vi "ControlMotorFindZeroEdge.vi"(2 "错误输入":errorcluster, 3 "控制电机":T1) -> (0 "错误输出":errorcluster)   [LabVIEW 2018]
panel:
  out "function return":i32
  out "搜零参数.搜零低速度":dbl
  out "搜零参数.搜零高速度":dbl
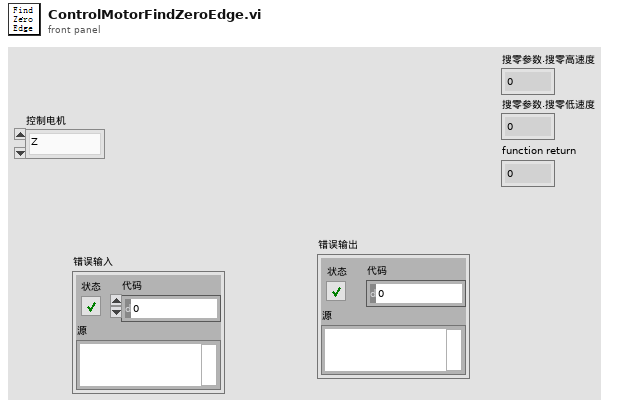
[diagram p1: front panel]
types:
  T1 = typedef "控制电机枚举器.ctl" = enum16{"Z", "Y", "X", "发散角", "俯仰", "旋转"}
  T2 = cluster{"是否停止":enum16{"解除停止", "停止"}, "发生错误停止运行":enum16{"不停止", "停止"}, "发生错误退出运行":enum16{"不退出", "退出"}, "有效电平":cluster{"脉冲信号有效电平":enum16{"低电平有效", "高电平有效"}, "方向信号有效电平 ":enum16{"低电平有效", "高电平有效"}}, "运行脉宽":i32, "加速度和速度边界":cluster{"加速度最大":i32, "速度最大":i32}, "硬件限位设置":cluster{"正限位使能":enum16{"不使能", "使能"}, "正限位极性":enum16{"低电平有效", "高电平有效"}, "负限位使能 ":enum16{"不使能", "使能"}, "负限位极性 ":enum16{"低电平有效", "高电平有效"}}, "伺服报警":cluster{"伺服报警使能":enum16{"不使能", "使能"}, "伺服报警极性":enum16{"低电平有效", "高电平有效"}}, "电机使能":enum16{"不使能", "使能"}, "输出极性":cluster{"寄存器":u32, " fifo":u32, "Bit":u32, "输出极性控制":enum16{"脉冲+方向", "正负脉冲"}}, "运动模式":enum16{"普通模式", "跟踪模式"}, "加速度 puls/s2":i32, "运动速度":cluster{"峰值速度 puls/s":i32, "起始速度puls/s":i32}, "电机速度归一化常量":dbl, "编码器":cluster{"编码器计数模式":enum16{"正交模式", "脉冲+方向模式"}, "编码器计数方向":enum16{"B相超前A相", "A相超前B相"}, "编码器使能":enum16{"不使能", "使能"}, "寄存器位置":i32, "fifo":i32, "data":i32}, "搜零参数":cluster{"orgSW零点开关":enum16{"0开关作为0点", "正限位作为0点", "负限位作为0点"}, "搜零方向":enum16{"正方向", "负方向"}, "零点停止方式":enum16{"立即停止", "减速停止"}, "原点信号边沿":enum16{"下降沿", "上升沿"}, "判断原点位置方向":enum16{"正方向移动", "负方向移动"}, " reducer搜零方式":enum16{"没有减速装置", "原点边缘作为减速", "探针开关作为减速"}, "零点位置":dbl, "搜零高速度":dbl, "搜零低速度":dbl, " 是否等待结束":enum16{"不等待", "等待"}, "编码器索引信号极性":enum16{"下降沿有效", "上升沿有效"}}}
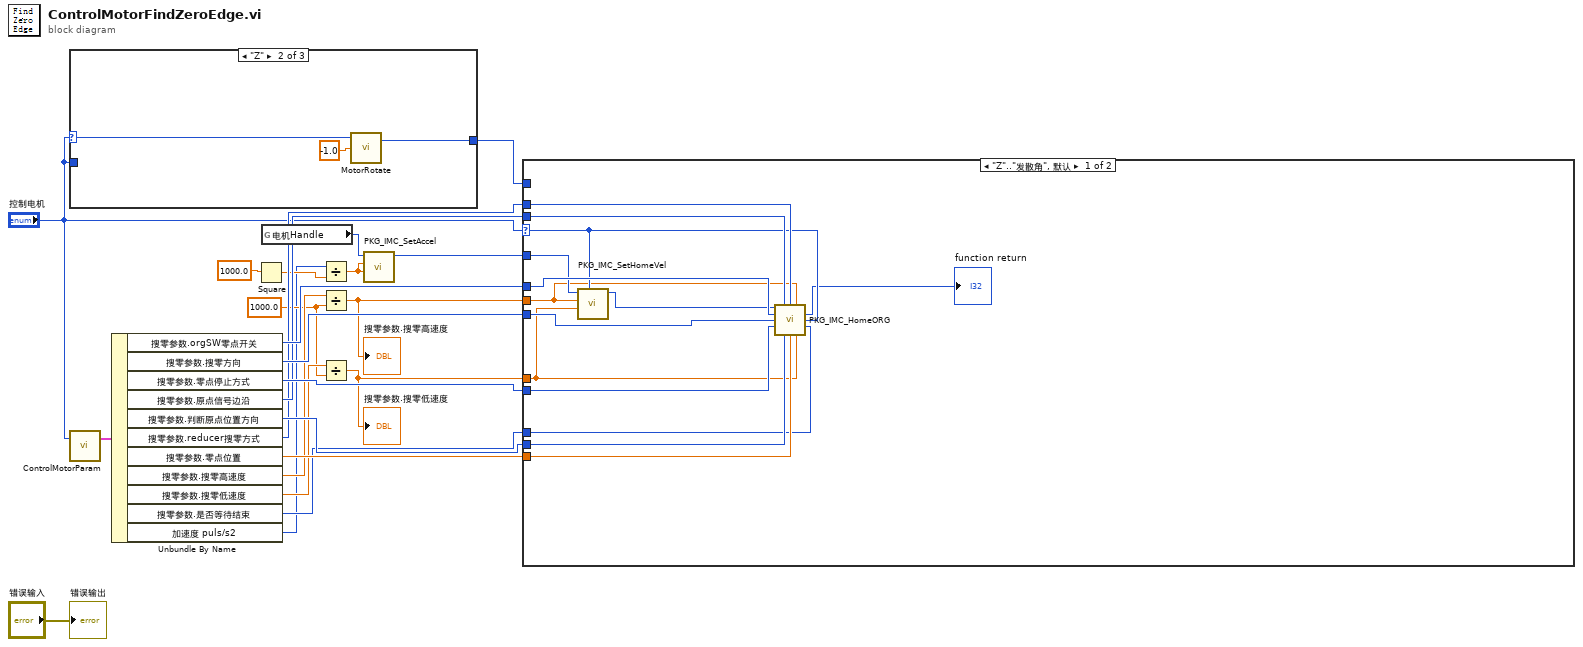
[diagram p0: block diagram]
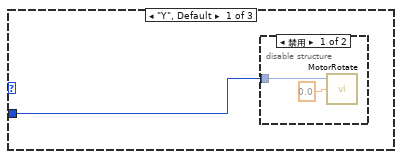
[diagram p2: hidden frame]
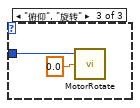
[diagram p4: hidden frame]
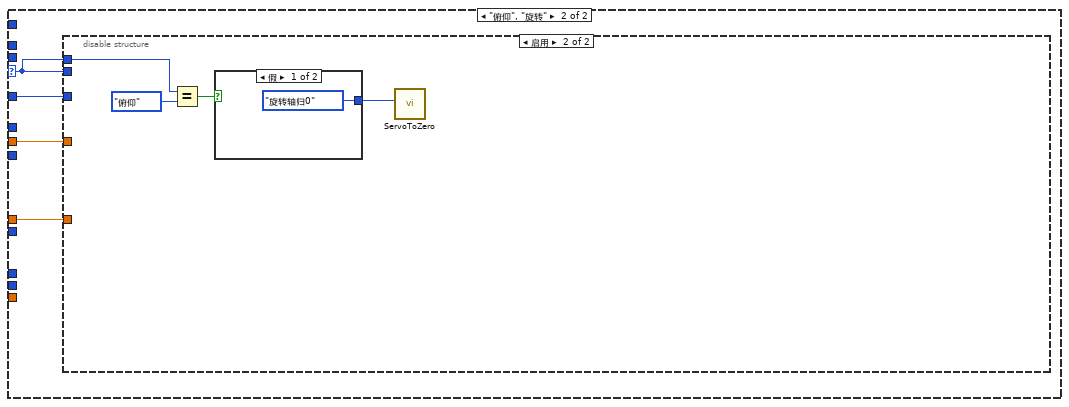
[diagram p5: hidden frame]
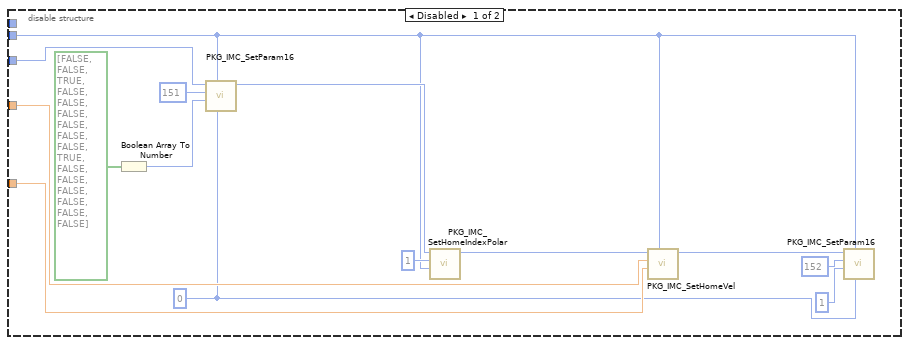
[diagram p6: hidden frame]
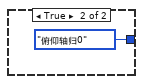
[diagram p7: hidden frame]
diagram:
  w8 = 1000.0 ("y")
  n1 = case shown="\"Z\"" "控制电机" {
    selector: "控制电机" -> [_ w29 _]
    tunnel: "控制电机" -> [w24 _ w30]
    tunnel: [_ w27 _] -> w7
    frame "Y", Default {
      n2 = disable-structure shown="禁用" {
        disable-tunnel: w24 -> [w25 _]
        frame Disabled {
          n3 = call "MotorRotate.vi"("位置"=0.0, "控制电机"=w25) -> ()  [unwired: 2 in, 1 out]
        }
        frame Enabled {
        }
      }
    }
    frame "Z" {
      n4 = call "MotorRotate.vi"("位置"=-1.0, "控制电机"=w29) -> ("返回"=w27:i32)  [unwired: 2 in]
    }
    frame "俯仰", "旋转" {
      n5 = call "MotorRotate.vi"("位置"=0.0, "控制电机"=w30) -> ()  [unwired: 2 in, 1 out]
    }
  }
  n6 = call "ControlMotorParam.vi"("控制电机"="控制电机") -> ("轴参数"=w11:T2)  [unwired: 2 in]
  n7 = Unbundle By Name(w11) -> ("搜零参数.orgSW零点开关"=w23:enum16{"0开关作为0点", "正限位作为0点", "负限位作为0点"}, "搜零参数.搜零方向"=w22:enum16{"正方向", "负方向"}, "搜零参数.零点停止方式"=w21:enum16{"立即停止", "减速停止"}, "搜零参数.原点信号边沿"=w20:enum16{"下降沿", "上升沿"}, "搜零参数.判断原点位置方向"=w19:enum16{"正方向移动", "负方向移动"}, "搜零参数.reducer搜零方式"=w18:enum16{"没有减速装置", "原点边缘作为减速", "探针开关作为减速"}, "搜零参数.零点位置"=w17:dbl, "搜零参数.搜零高速度"=w10:dbl, "搜零参数.搜零低速度"=w9:dbl, "搜零参数.是否等待结束"=w16:enum16{"不等待", "等待"}, "加速度 puls/s2"=w1:i32)
  n8 = Square(x=1000.0) -> (x^2=w4:dbl)
  n9 = global read "参数.vi" "电机Handle"() -> (w3:u32)
  n10 = Divide(x=w1, y=w4) -> (x/y=w6:dbl)
  n11 = Divide(x=w10, y=w8) -> (x/y=w15:dbl)
  "搜零参数.搜零高速度" <- w15
  n12 = Divide(x=w9, y=w8) -> (x/y=w14:dbl)
  "搜零参数.搜零低速度" <- w14
  n13 = call "PKG_IMC_SetAccel.vi"("decel"=w6, "accel"=w6, "handle"=w3) -> ("handle out"=w2:u32)  [unwired: 7 in, 1 out]
  n14 = case shown="\"Z\"..\"发散角\", 默认" "控制电机" {
    selector: "控制电机" -> [w35 w46]
    tunnel: w23 -> [w45 _]
    tunnel: w22 -> [w44 _]
    tunnel: w21 -> [w43 _]
    tunnel: w20 -> [w42 _]
    tunnel: w19 -> [w41 _]
    tunnel: w18 -> [w40 _]
    tunnel: w17 -> [w39 _]
    tunnel: w15 -> [w34 w48]
    tunnel: w14 -> [w33 w47]
    tunnel: w16 -> [w38 _]
    tunnel: w2 -> [w36 w49]
    tunnel: w7 -> [_ _]
    frame "Z".."发散角", Default {
      n15 = call "PKG_IMC_SetHomeVel.vi"("axis"=w35, "low"=w33, "hight"=w34, "handle"=w36) -> ("handle out"=w37:u32)  [unwired: 6 in, 1 out]
      n16 = call "PKG_IMC_HomeORG.vi"("Handle"=w37, "riseEdge"=w42, "reducer"=w40, "hightvel"=w34, "orgSW"=w45, "dir"=w44, "axis"=w35, "stopmode"=w43, "wait"=w38, "edir"=w41, "pos"=w39, "lowvel"=w33) -> ("function return"=→"function return":i32)  [unwired: 2 in, 1 out]
    }
    frame "俯仰", "旋转" {
      n17 = disable-structure shown="启用" {
        disable-tunnel: w49 -> [w63 _]
        disable-tunnel: w48 -> [w59 _]
        disable-tunnel: w47 -> [w58 _]
        disable-tunnel: w46 -> [w50 _]
        disable-tunnel: w46 -> [_ w67]
        frame Disabled {
          w56 = 0 ("fifo")
          n18 = Boolean Array To Number(Boolean array=bool[] [FALSE, FALSE, TRUE, FALSE, FALSE, FALSE, FALSE, FALSE, FALSE, TRUE, FALSE, FALSE, FALSE, FALSE, FALSE, FALSE] ("布尔数组")) -> (number=w61:u32)
          n19 = call "PKG_IMC_SetParam16.vi"("fifo"=w56, "axis"=w50, "data"=w61, "paramloc"=i16 151, "Handle"=w63) -> ("Handle out"=w53:u32)  [unwired: 5 in, 1 out]
          n20 = call "PKG_IMC_SetHomeIndexPolar.vi"("axis"=w50, "polar"=1, "handle"=w53) -> ("handle out"=w52:u32)  [unwired: 7 in, 1 out]
          n21 = call "PKG_IMC_SetHomeVel.vi"("axis"=w50, "low"=w58, "hight"=w59, "handle"=w52) -> ("handle out"=w57:u32)  [unwired: 6 in, 1 out]
          n22 = call "PKG_IMC_SetParam16.vi"("fifo"=w56, "axis"=w50, "data"=i16 1, "paramloc"=i16 152, "Handle"=w57) -> ()  [unwired: 5 in, 2 out]
        }
        frame Enabled {
          n23 = Equal?(x=w67, y=控制电机枚举器."俯仰") -> (x = y?=w65:bool)
          n24 = case shown="假" w65 {
            tunnel: [enum16{"俯仰轴归0", "旋转轴归0", "空"}."旋转轴归0" ("动作IO") enum16{"俯仰轴归0", "旋转轴归0", "空"}."俯仰轴归0" ("动作IO")] -> w64
            frame False {
            }
            frame True {
            }
          }
          n25 = call "ServoToZero.vi"("动作IO"=w64) -> ()  [unwired: 11 in]
        }
      }
    }
  }
  "错误输出" <- "错误输入"
